vi "VI Tree - Python Data Tools.vi"   [LabVIEW 2020]
uses:
  LabVIEW Data to Python String/LabVIEW Data to Python String (U64).vi
  Python String to LabVIEW Data/Python String to LabVIEW Data (Variant).vi
  jki_python_data_tools.lvlib
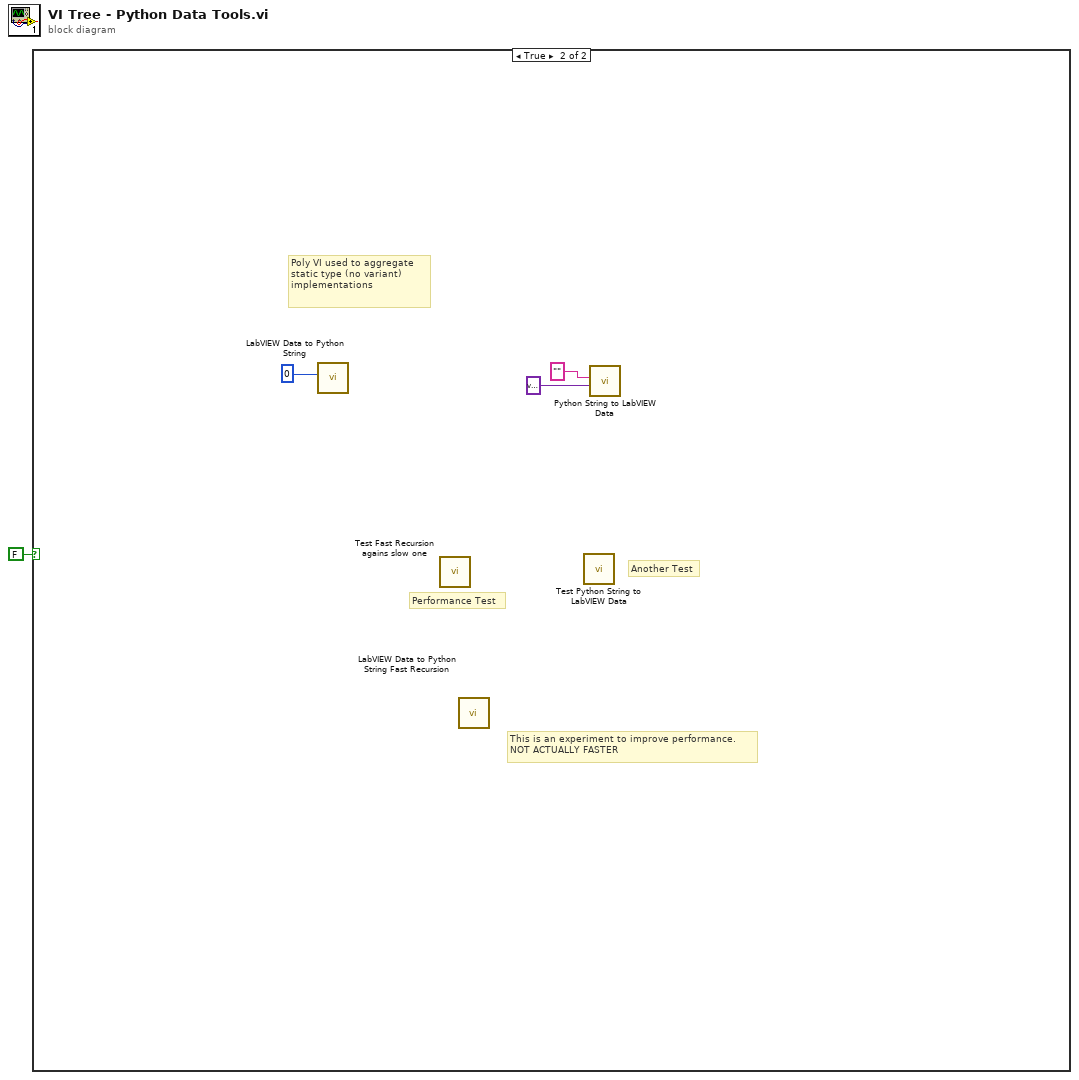
[diagram p0: block diagram]
diagram:
  n1 = case shown="True" FALSE {
    frame False {
    }
    frame True {
      # "Poly VI used to aggregate static type (no variant) implementations"
      # "Another Test"
      # "Performance Test"
      # "This is an experiment to improve performance.\nNOT ACTUALLY FASTER"
      n2 = call-poly "LabVIEW Data to Python String.vi"("LabVIEW Data"=u64 0) -> ()  [unwired: 9 in, 2 out]
      n3 = call "Test Fast Recursion agains slow one.vi"() -> ()  [unwired: 1 in]
      n4 = call "LabVIEW Data to Python String Fast Recursion.vi"() -> ()  [unwired: 10 in, 2 out]
      n5 = call "Test Python String to LabVIEW Data.vi"() -> ()  [unwired: 1 in]
      n6 = call-poly "Python String to LabVIEW Data.vi"("type"=variant, "Python String"="") -> ()  [unwired: 8 in, 2 out]
    }
  }
